vi "Wait on VI to Execute.vi"(8 "error in (no error)":errorcluster, 10 "VI Refnum in":refnum<vi>, 11 "Slave Test Runner in":refnum<class "Slave Test Runner.lvclass">) -> (0 "error out":errorcluster, 2 "VI Refnum out":refnum<vi>, 3 "Slave Test Runner out":refnum<class "Slave Test Runner.lvclass">)   [LabVIEW 2020, in "Slave Test Runner.lvclass"]
uses:
  Slave Test Runner.lvclass
  Slave Test Runner.lvclass/Slave Test Runner.ctl
  <vilib>/Utility/error.llb/Error Cluster From Error Code.vi
  <vilib>/ErrorRing/Error Ring.xnode
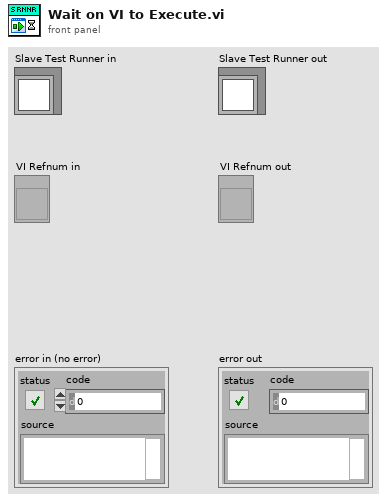
[diagram p1: front panel]
types:
  T1 = enum32{"Bad", "Idle", "Run top level", "Running"}
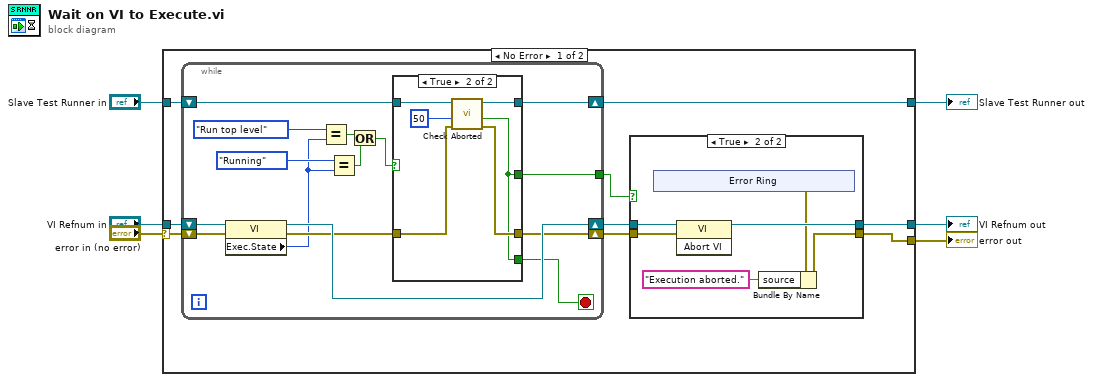
[diagram p0: block diagram]
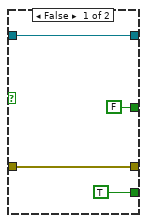
[diagram p3: hidden frame]
diagram:
  n1 = case shown="No Error" "error in (no error)" {
    selector: "error in (no error)" -> [w13 w55]
    tunnel: [w15 w53] -> w6
    tunnel: "Slave Test Runner in" -> [w14 w53]
    tunnel: "VI Refnum in" -> [w11 w54]
    tunnel: [w10 w54] -> w2
    tunnel: [w8 w55] -> w1
    frame No Error {
      n2 = while {
        shift-right: [w42] -> w15
        shift-left: w14 -> [w41]
        shift-right: [w35] -> w9
        shift-left: w13 -> [w40]
        shift-right: [w39] -> w12
        shift-left: w11 -> [w38]
        tunnel: [w34] -> w7
        stop <- w32 stop-if-true
        n3 = property class="VI"(reference=w38, error in=w40) -> (reference out=w39:refnum<vi>, error out=w36:errorcluster, "Exec.State"=w28:T1)
        n4 = Equal?(x=T1."Run top level" ("Execution:State"), y=w28) -> (x = y?=w29:bool)
        n5 = Equal?(x=T1."Running" ("Execution:State"), y=w28) -> (x = y?=w33:bool)
        n6 = Or(x=w29, y=w33) -> (x .or. y?=w30:bool)
        n7 = case shown="True" w30 {
          tunnel: [w46 w52] -> w42
          tunnel: w41 -> [w46 w51]
          tunnel: w36 -> [w44 w49]
          tunnel: [w44 w48] -> w35
          tunnel: [FALSE ("Aborted?") w47] -> w34
          tunnel: [TRUE ("Aborted?") w47] -> w32
          frame False {
          }
          frame True {
            n8 = call "Check Aborted.vi"("error in (no error)"=w49, "timeout in ms (0)"=50, "Slave Test Runner In"=w51) -> ("error out"=w48:errorcluster, "Aborted?"=w47:bool, "Slave Test Runner Out"=w52:refnum<class "Slave Test Runner.lvclass">)  [unwired: 6 in]
          }
        }
      }
      n9 = case shown="True" w7 {
        tunnel: w12 -> [w17 w23]
        tunnel: [w17 w22] -> w10
        tunnel: w9 -> [w16 w21]
        tunnel: [w16 w19] -> w8
        frame False {
        }
        frame True {
          n10 = xnode "Error Ring"() -> ("error out"=w20:errorcluster)
          n11 = invoke class="VI" method="Abort VI"(reference=w23, error in=w21) -> (reference out=w22:refnum<vi>)  [unwired: 1 in, 2 out]
          n12 = Bundle By Name(cluster=w20, "source"="Execution aborted.") -> (w19:errorcluster)
        }
      }
    }
    frame Error {
    }
  }
  "Slave Test Runner out" <- w6
  "error out" <- w1
  "VI Refnum out" <- w2
